vi "Final_OCVACIR.vi"(10 "Cluster":T1, 11 "L2T":T2) -> (2 "Boolean":bool, 3 "Boolean 2":bool)   [LabVIEW 2020]
uses:
  Ctrl/L2T.ctl
panel:
  # "Pre DCIR_____________________________________"
  # "intra DCIR_____________________________________"
  # "Post DCIR_____________________________________"
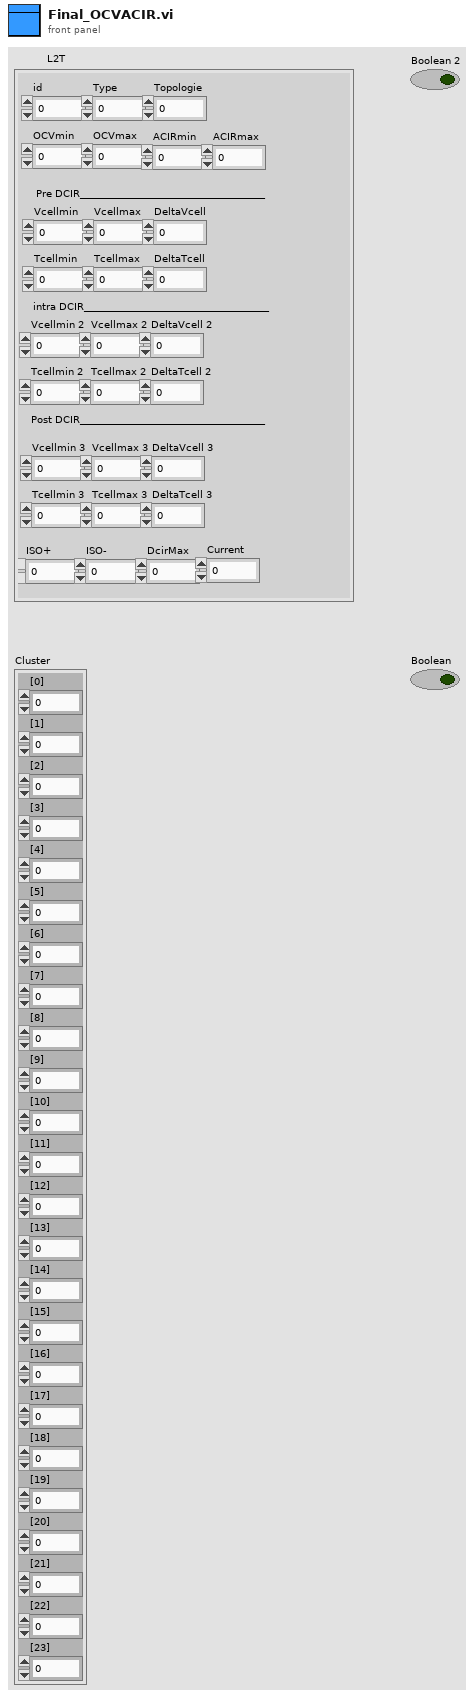
[diagram p1: front panel]
types:
  T1 = cluster{"[0]":dbl, "[1]":dbl, "[2]":dbl, "[3]":dbl, "[4]":dbl, "[5]":dbl, "[6]":dbl, "[7]":dbl, "[8]":dbl, "[9]":dbl, "[10]":dbl, "[11]":dbl, "[12]":dbl, "[13]":dbl, "[14]":dbl, "[15]":dbl, "[16]":dbl, "[17]":dbl, "[18]":dbl, "[19]":dbl, "[20]":dbl, "[21]":dbl, "[22]":dbl, "[23]":dbl}
  T2 = typedef "L2T.ctl" = cluster{"id":dbl, "Type":dbl, "OCVmin":dbl, "OCVmax":dbl, "ACIRmin":dbl, "ACIRmax":dbl, "Vcellmin":dbl, "Vcellmax":dbl, "DeltaVcell":dbl, "Tcellmin":dbl, "Tcellmax":dbl, "DeltaTcell":dbl, "ISO+":dbl, "ISO-":dbl, "DcirMax":dbl, "Current":dbl, "Topologie":dbl, "Vcellmin 2":dbl, "Vcellmax 2":dbl, "DeltaVcell 2":dbl, "Tcellmin 2":dbl, "Tcellmax 2":dbl, "DeltaTcell 2":dbl, "Vcellmin 3":dbl, "Vcellmax 3":dbl, "DeltaVcell 3":dbl, "Tcellmin 3":dbl, "Tcellmax 3":dbl, "DeltaTcell 3":dbl}
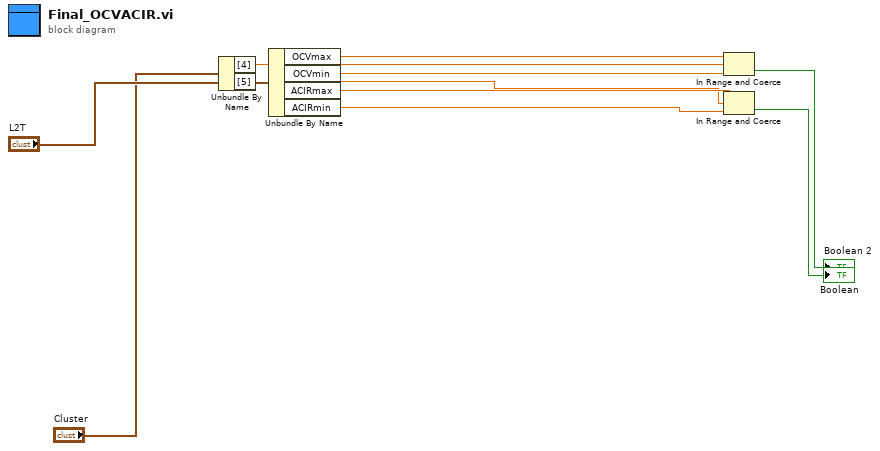
[diagram p0: block diagram]
diagram:
  n1 = Unbundle By Name("Cluster") -> ("[4]"=w4:dbl, "[5]"=w5:dbl)
  n2 = Unbundle By Name("L2T") -> ("OCVmax"=w7:dbl, "OCVmin"=w8:dbl, "ACIRmax"=w9:dbl, "ACIRmin"=w10:dbl)
  n3 = In Range and Coerce(upper limit=w7, x=w4, lower limit=w8) -> (In Range?=→"Boolean 2":bool)  [unwired: 1 out]
  n4 = In Range and Coerce(upper limit=w9, x=w5, lower limit=w10) -> (In Range?=→"Boolean":bool)  [unwired: 1 out]
